vi "9.5.vi"() -> ()   [LabVIEW 2019]
panel:
  out "?":string
  out "kansen":dbl
  in  "invoer":dbl
  # "getal tussen de 1 en 10"
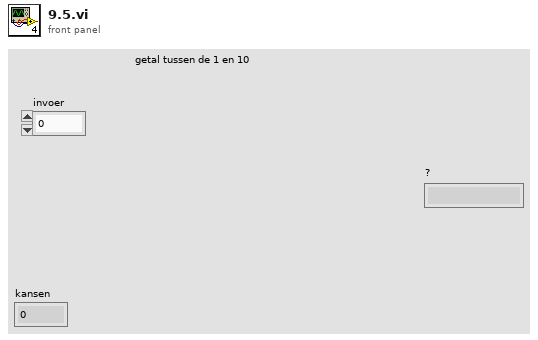
[diagram p1: front panel]
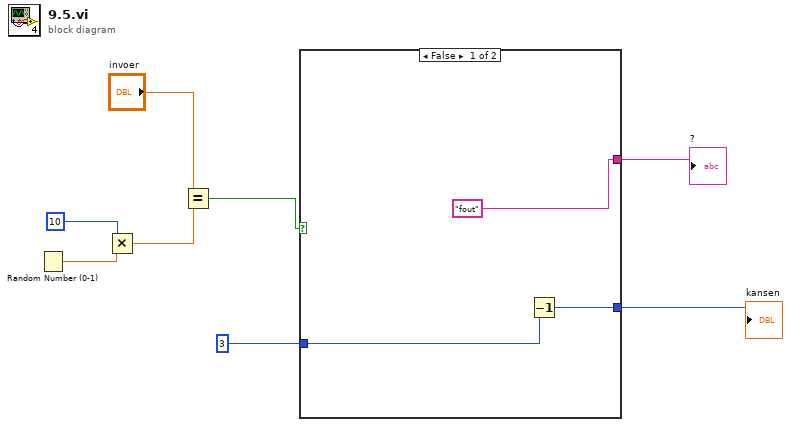
[diagram p0: block diagram]
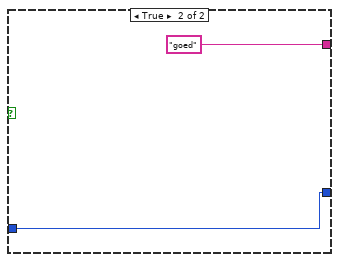
[diagram p2: hidden frame]
diagram:
  n1 = Random Number (0-1)() -> (number: 0 to 1=w3:dbl)
  n2 = Multiply(x=10, y=w3) -> (x*y=w1:dbl)
  n3 = Equal?(x="invoer", y=w1) -> (x = y?=w7:bool)
  n4 = case shown="False" w7 {
    tunnel: ["fout" "goed"] -> w6
    tunnel: 3 -> [w10 w12]
    tunnel: [w9 w12] -> w4
    frame False {
      n5 = Decrement(x=w10) -> (x-1=w9:i32)
    }
    frame True {
    }
  }
  "kansen" <- w4
  "?" <- w6
